vi "create data FIFOs.vi"(7 "FIFO name prefix":string, 8 "error in (no error)":errorcluster, 11 "counts":T3[](array[typedef])) -> (0 "error out":errorcluster, 2 "Requested Types":T1[](array[typedef]), 3 "Data FIFOs":T2)   [LabVIEW 2015, in "E2E Runtime (RT FIFO).lvclass"]
uses:
  E2E Runtime (RT FIFO).lvclass
  <vilib>/NI/Tag Bus/table/allocation specification.ctl
  <vilib>/NI/Tag Bus/tag/Data Type.ctl
  Data FIFOs.ctl
  <vilib>/Utility/error.llb/Error Cluster From Error Code.vi
  <vilib>/ErrorRing/Error Ring.xnode
  <vilib>/NI/Tag Bus/tag/tag descriptor.lvclass
  <vilib>/NI/Tag Bus/table/data table.lvlib
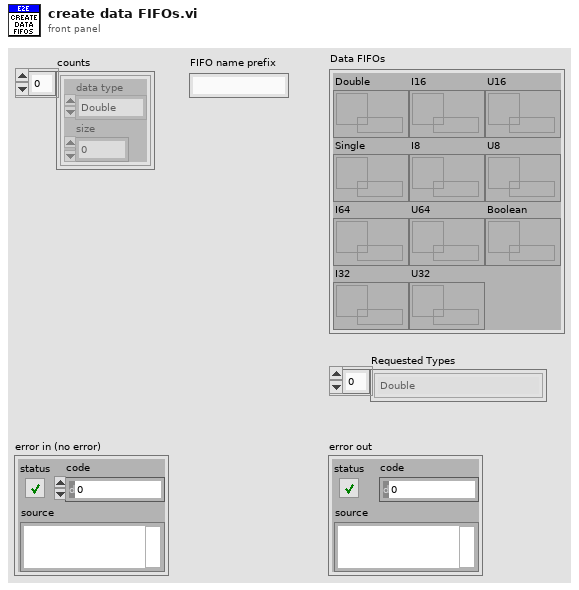
[diagram p1: front panel]
types:
  T1 = typedef "tag bus.lvlib/tag descriptor.lvclass/Data Type.ctl" = enum16{"Double", "Single", "I64", "I32", "I16", "I8", "U64", "U32", "U16", "U8", "Boolean", "String", "Array of Double", "Array of Single", "Array of I64", "Array of I32", "Array of I16", "Array of I8", "Array of U64", "Array of U32", "Array of U16", "Array of U8", "Array of Boolean", "Array of String"}
  T2 = typedef "E2E Runtime (RT FIFO).lvclass/Data FIFOs.ctl" = cluster{"Double":refnum<k33>, "Single":refnum<k33>, "I64":refnum<k33>, "I32":refnum<k33>, "I16":refnum<k33>, "I8":refnum<k33>, "U64":refnum<k33>, "U32":refnum<k33>, "U16":refnum<k33>, "U8":refnum<k33>, "Boolean":refnum<k33>}
  T3 = typedef "tag bus.lvlib/data table.lvlib/allocation specification.ctl" = cluster{"data type":T1, "size":i32}
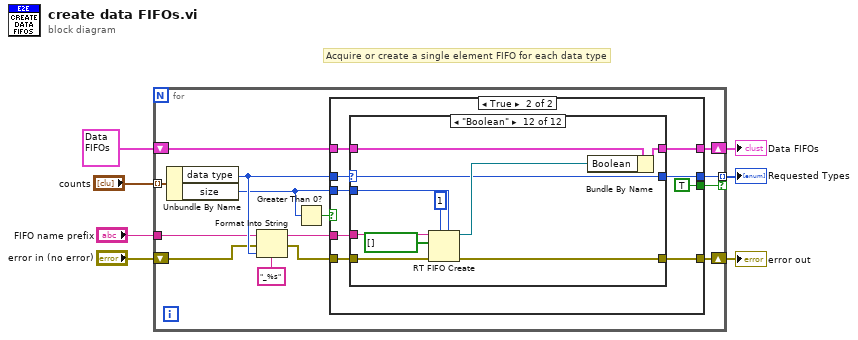
[diagram p0: block diagram]
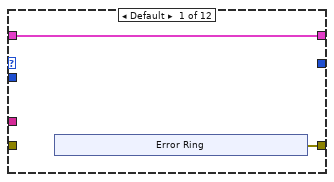
[diagram p3: hidden frame]
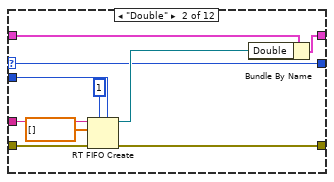
[diagram p4: hidden frame]
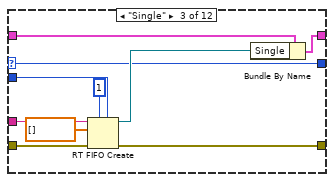
[diagram p5: hidden frame]
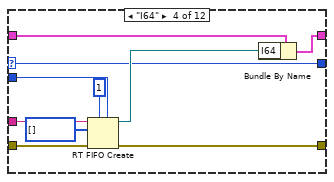
[diagram p6: hidden frame]
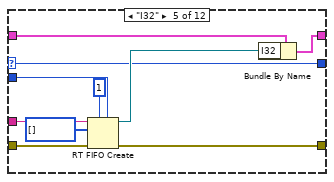
[diagram p7: hidden frame]
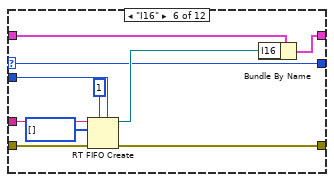
[diagram p8: hidden frame]
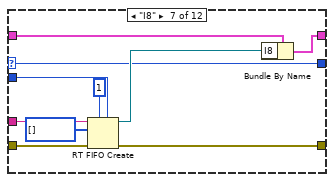
[diagram p9: hidden frame]
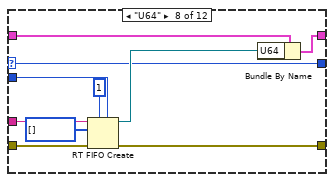
[diagram p10: hidden frame]
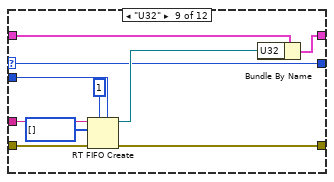
[diagram p11: hidden frame]
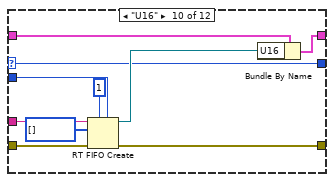
[diagram p12: hidden frame]
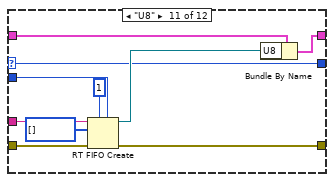
[diagram p13: hidden frame]
diagram:
  # "Acquire or create a single element FIFO for each data type"
  n1 = for {
    tunnel: "counts" -> [w21] mode=indexing
    shift-right: [w18] -> w3
    shift-left: "error in (no error)" -> [w14]
    shift-right: [w19] -> w4
    shift-left: T2 {"Double"=refnum, "Single"=refnum, "I64"=refnum, "I32"=refnum, "I16"=refnum, "I8"=refnum, "U64"=refnum, "U32"=refnum, "U16"=refnum, "U8"=refnum, "Boolean"=refnum} ("Cluster") -> [w20]
    tunnel: "FIFO name prefix" -> [w16]
    tunnel: [w9] -> w1 mode=indexing if=w8
    n2 = Unbundle By Name(w21) -> ("data type"=w17:T1, "size"=w11:i32)
    n3 = Format Into String(format string="_%s", initial string=w16, error in=w14, w17) -> (resulting string=w15:string, error out=w13:errorcluster)
    n4 = Greater Than 0?(x=w11) -> (x > 0?=w10:bool)
    n5 = case shown="True" w10 {
      tunnel: w20 -> [w23 w32]
      tunnel: [w23 w31] -> w19
      tunnel: [w22 w30] -> w18
      tunnel: w17 -> [_ w29]
      tunnel: w15 -> [_ w28]
      tunnel: w13 -> [w22 w27]
      tunnel: w11 -> [_ w26]
      tunnel: [_ w25] -> w9
      tunnel: [_ TRUE] -> w8
      frame False {
      }
      frame True {
        n6 = case shown="\"Boolean\"" w29 {
          selector: w29 -> [_ w39 w49 w59 w69 w79 w89 w99 w109 w119 w129 w139]
          tunnel: w26 -> [_ w47 w57 w67 w77 w87 w97 w107 w117 w127 w137 w147]
          tunnel: w27 -> [_ w48 w58 w68 w78 w88 w98 w108 w118 w128 w138 w148]
          tunnel: w32 -> [w34 w45 w55 w65 w75 w85 w95 w105 w115 w125 w135 w145]
          tunnel: [w34 w43 w53 w63 w73 w83 w93 w103 w113 w123 w133 w143] -> w31
          tunnel: [w33 w42 w52 w62 w72 w82 w92 w102 w112 w122 w132 w142] -> w30
          tunnel: w28 -> [_ w40 w50 w60 w70 w80 w90 w100 w110 w120 w130 w140]
          tunnel: [_ w39 w49 w59 w69 w79 w89 w99 w109 w119 w129 w139] -> w25
          frame Default {
            n7 = xnode "Error Ring"() -> ("error out"=w33:errorcluster)
          }
          frame "Double" {
            n8 = RT FIFO Create(0:w40, 1:dbl[] [], 3:w48, 4:u32 1 ("size (10)"), 6:w47) -> (8:w44:refnum<k33>, 11:w42:errorcluster)  [unwired: 3 in, 1 out]
            n9 = Bundle By Name(cluster=w45, "Double"=w44) -> (w43:T2)
          }
          frame "Single" {
            n10 = RT FIFO Create(0:w50, 1:sgl[] [], 3:w58, 4:u32 1 ("size (10)"), 6:w57) -> (8:w54:refnum<k33>, 11:w52:errorcluster)  [unwired: 3 in, 1 out]
            n11 = Bundle By Name(cluster=w55, "Single"=w54) -> (w53:T2)
          }
          frame "I64" {
            n12 = RT FIFO Create(0:w60, 1:i64[] [], 3:w68, 4:u32 1 ("size (10)"), 6:w67) -> (8:w64:refnum<k33>, 11:w62:errorcluster)  [unwired: 3 in, 1 out]
            n13 = Bundle By Name(cluster=w65, "I64"=w64) -> (w63:T2)
          }
          frame "I32" {
            n14 = RT FIFO Create(0:w70, 1:i32[] [], 3:w78, 4:u32 1 ("size (10)"), 6:w77) -> (8:w74:refnum<k33>, 11:w72:errorcluster)  [unwired: 3 in, 1 out]
            n15 = Bundle By Name(cluster=w75, "I32"=w74) -> (w73:T2)
          }
          frame "I16" {
            n16 = RT FIFO Create(0:w80, 1:i16[] [], 3:w88, 4:u32 1 ("size (10)"), 6:w87) -> (8:w84:refnum<k33>, 11:w82:errorcluster)  [unwired: 3 in, 1 out]
            n17 = Bundle By Name(cluster=w85, "I16"=w84) -> (w83:T2)
          }
          frame "I8" {
            n18 = RT FIFO Create(0:w90, 1:i8[] [], 3:w98, 4:u32 1 ("size (10)"), 6:w97) -> (8:w94:refnum<k33>, 11:w92:errorcluster)  [unwired: 3 in, 1 out]
            n19 = Bundle By Name(cluster=w95, "I8"=w94) -> (w93:T2)
          }
          frame "U64" {
            n20 = RT FIFO Create(0:w100, 1:u64[] [], 3:w108, 4:u32 1 ("size (10)"), 6:w107) -> (8:w104:refnum<k33>, 11:w102:errorcluster)  [unwired: 3 in, 1 out]
            n21 = Bundle By Name(cluster=w105, "U64"=w104) -> (w103:T2)
          }
          frame "U32" {
            n22 = RT FIFO Create(0:w110, 1:u32[] [], 3:w118, 4:u32 1 ("size (10)"), 6:w117) -> (8:w114:refnum<k33>, 11:w112:errorcluster)  [unwired: 3 in, 1 out]
            n23 = Bundle By Name(cluster=w115, "U32"=w114) -> (w113:T2)
          }
          frame "U16" {
            n24 = RT FIFO Create(0:w120, 1:u16[] [], 3:w128, 4:u32 1 ("size (10)"), 6:w127) -> (8:w124:refnum<k33>, 11:w122:errorcluster)  [unwired: 3 in, 1 out]
            n25 = Bundle By Name(cluster=w125, "U16"=w124) -> (w123:T2)
          }
          frame "U8" {
            n26 = RT FIFO Create(0:w130, 1:u8[] [], 3:w138, 4:u32 1 ("size (10)"), 6:w137) -> (8:w134:refnum<k33>, 11:w132:errorcluster)  [unwired: 3 in, 1 out]
            n27 = Bundle By Name(cluster=w135, "U8"=w134) -> (w133:T2)
          }
          frame "Boolean" {
            n28 = RT FIFO Create(0:w140, 1:bool[] [], 3:w148, 4:u32 1 ("size (10)"), 6:w147) -> (8:w144:refnum<k33>, 11:w142:errorcluster)  [unwired: 3 in, 1 out]
            n29 = Bundle By Name(cluster=w145, "Boolean"=w144) -> (w143:T2)
          }
        }
      }
    }
  }
  "Data FIFOs" <- w4
  "error out" <- w3
  "Requested Types" <- w1
